vi "GUI_laptop v11c2.vi"() -> ()   [LabVIEW 2019]
uses:
  <vilib>/Math Plots/3D Math Plots/3D Scatter/3D Scatter XCtrl/3D Scatter.xctl
  <vilib>/Platform/TimedLoop/XDataNode/timing_clust.ctl
  <vilib>/Platform/TimedLoop/XDataNode/nitl_modes.ctl
  <vilib>/Platform/TimedLoop/XDataNode/wakeup.ctl
  <vilib>/Analysis/_algsub.llb/Real Vector Norm.vi
  <vilib>/Instr/_visa.llb/VISA Configure Serial Port (Instr).vi
  <vilib>/Utility/file.llb/Write Delimited Spreadsheet (DBL).vi
  <vilib>/Math Plots/3D Math Plots/3D Scatter/3D Scatter Datatype/Public/Plot Helper (Vector).vi
  <vilib>/platform/TimedLoop/XDataNode/XDataNode.xnode
  <vilib>/Platform/TimedLoop/XDataNode/XDNodeRunTimeDep.lvlib
  <vilib>/Analysis/NI_AALPro.lvlib
  <vilib>/Math Plots/3D Math Plots/3D Scatter/3D Scatter Datatype/3D Scatter Datatype.lvclass
panel:
  in  "L5 Scale":dbl=330.0
  in  "L5 Upper Bound":dbl=330.0
  in  "L5 Lower Bound":dbl=320.0
  in  "Motion Scale 4":dbl=2.0
  out "spreadsheet string":string
  out "1-D Array of Real 2":dbl[](array[numeric])
  out "1-D Array of Real":dbl[](array[numeric])
  in  "Save Path 2":path=path "C:/Users/jimmy/Documents/GitHub/Arduino-LabVIEW/zhantao/read_data_delt.csv"
  out "Numeric":i32
  out "send values":dbl[](array[numeric])
  out "Robot Feedback (xyz)":dbl[](array[numeric])
  in  "UDP Send":bool
  in  "UDP Recv":bool
  in  "L5 bound":dbl=1000.0
  in  "L4 bound (deg)":dbl=1000.0
  in  "L3 bound (mm)":dbl=1000.0
  in  "L2 bound (deg)":dbl=1000.0
  in  "L1 bound (deg)":dbl=1000.0
  in  "Joystick Type":dbl(ring) items=["Rigid Joystick", "Free Joystick"]
  out "Finished Late? [i-1]":bool
  in  "Epsilon":dbl=0.2
  out "3D Scatter":refnum<class "3D Plot Datatype.lvclass">[](xcontrol)
  out "Random Point":dbl[](array[numeric])
  out "Virtual Cursor":dbl[](array[numeric])
  out "Iteration Duration":i64
  in  "Num of Points":i32=10
  in  "z bound":dbl=2.0
  in  "y bound":dbl=5.0
  in  "x bound":dbl=5.0
  in  "Stop":bool
  in  "Round Decimals":dbl=2.0 format="%#_15g"
  in  "Save  Data":bool
  in  "Save Path":path=path "C:/Users/jimmy/Documents/GitHub/Arduino-LabVIEW/zhantao/read_data_abs.csv"
  in  "x speed":dbl=0.5
  in  "z speed":dbl=0.5
  in  "y speed":dbl=0.5
  out "error out":errorcluster
  in  "baud rate":u32=115200
  in  "VISA resource name":refnum<visa-resource-name>
  # "TODO: fix the bounds; currently bounds are arbitrary"
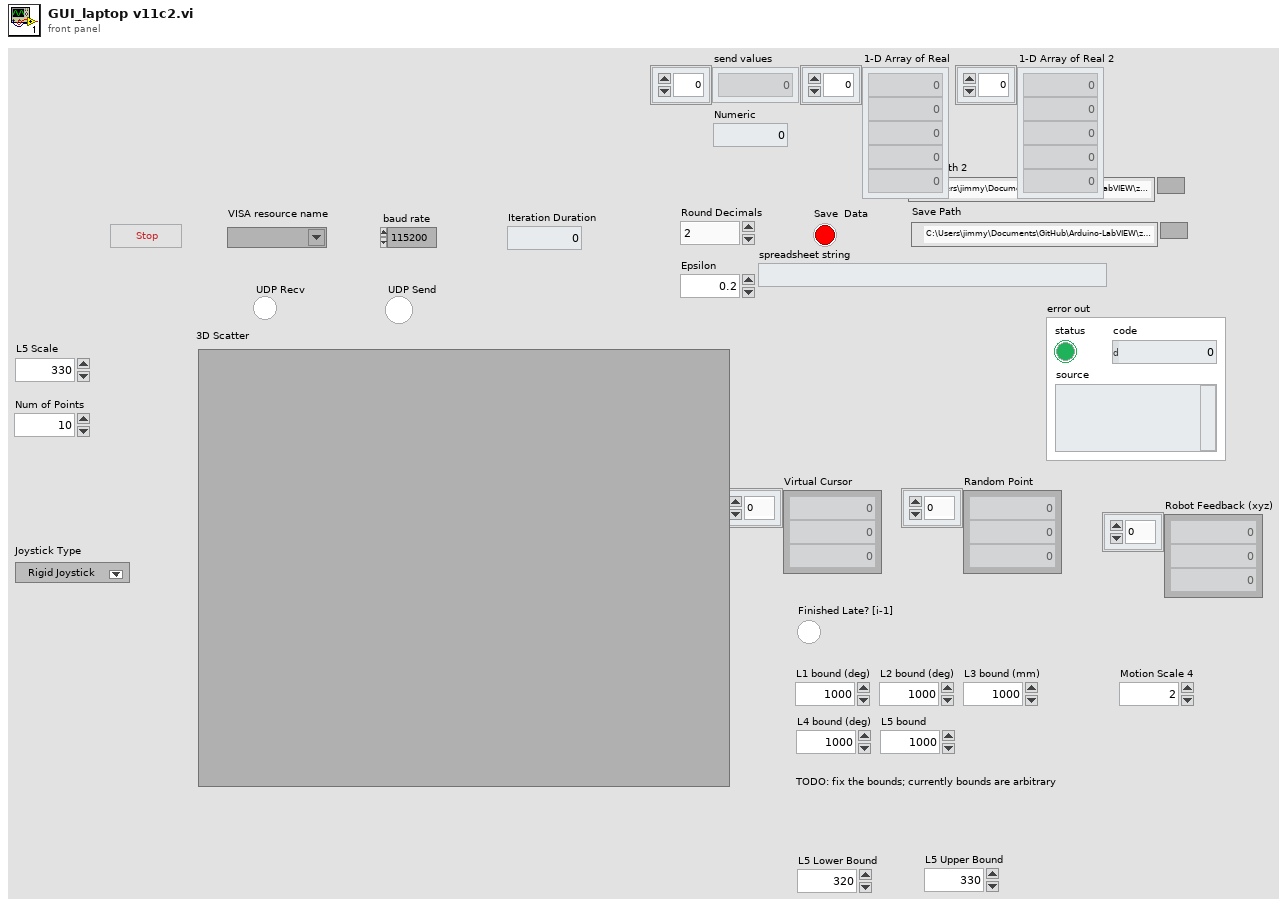
[diagram p1: front panel]
types:
  T1 = typedef "XDNodeRunTimeDep.lvlib/timing_clust.ctl" = cluster{"Expected End [f-1]":u64, "Actual End [f-1]":u64, "Finished Late? [f-1]":bool, "Expected End [i-1]":u64, "Actual End [i-1]":u64, "Finished Late? [i-1]":bool, "Expected Start [i]":u64, "Actual Start [i]":u64, "Expected Start [f]":u64, "Actual Start [f]":u64, "Source Name":string, "Structure Name":string, "Period":i64, "Deadline":i64, "Offset":i64, "Start":i64, "Priority":i32, "Timeout":i32, "Mode":T2, "Wakeup Reason":T3, "Error":errorcluster, "Source Type":string, "Secondary Source Type":string, "Global End Time":u64, "Global Start Time":u64, "Frame Duration":u64, "Iteration Duration":u64, "Assigned CPU":i32, "I/O Scan Engine Mode":u32}
  T2 = typedef "XDNodeRunTimeDep.lvlib/nitl_modes.ctl" = enum32{"No Change", "Process missed periods, maintain original phase", "Discard missed periods, maintain original phase", "Process missed periods, ignore original phase", "Discard missed periods, ignore original phase"}
  T3 = typedef "XDNodeRunTimeDep.lvlib/wakeup.ctl" = enum32{"Normal", "Aborted", "Asynchronous wakeup", "Timing source error", "Timed loop error", "Timeout"}
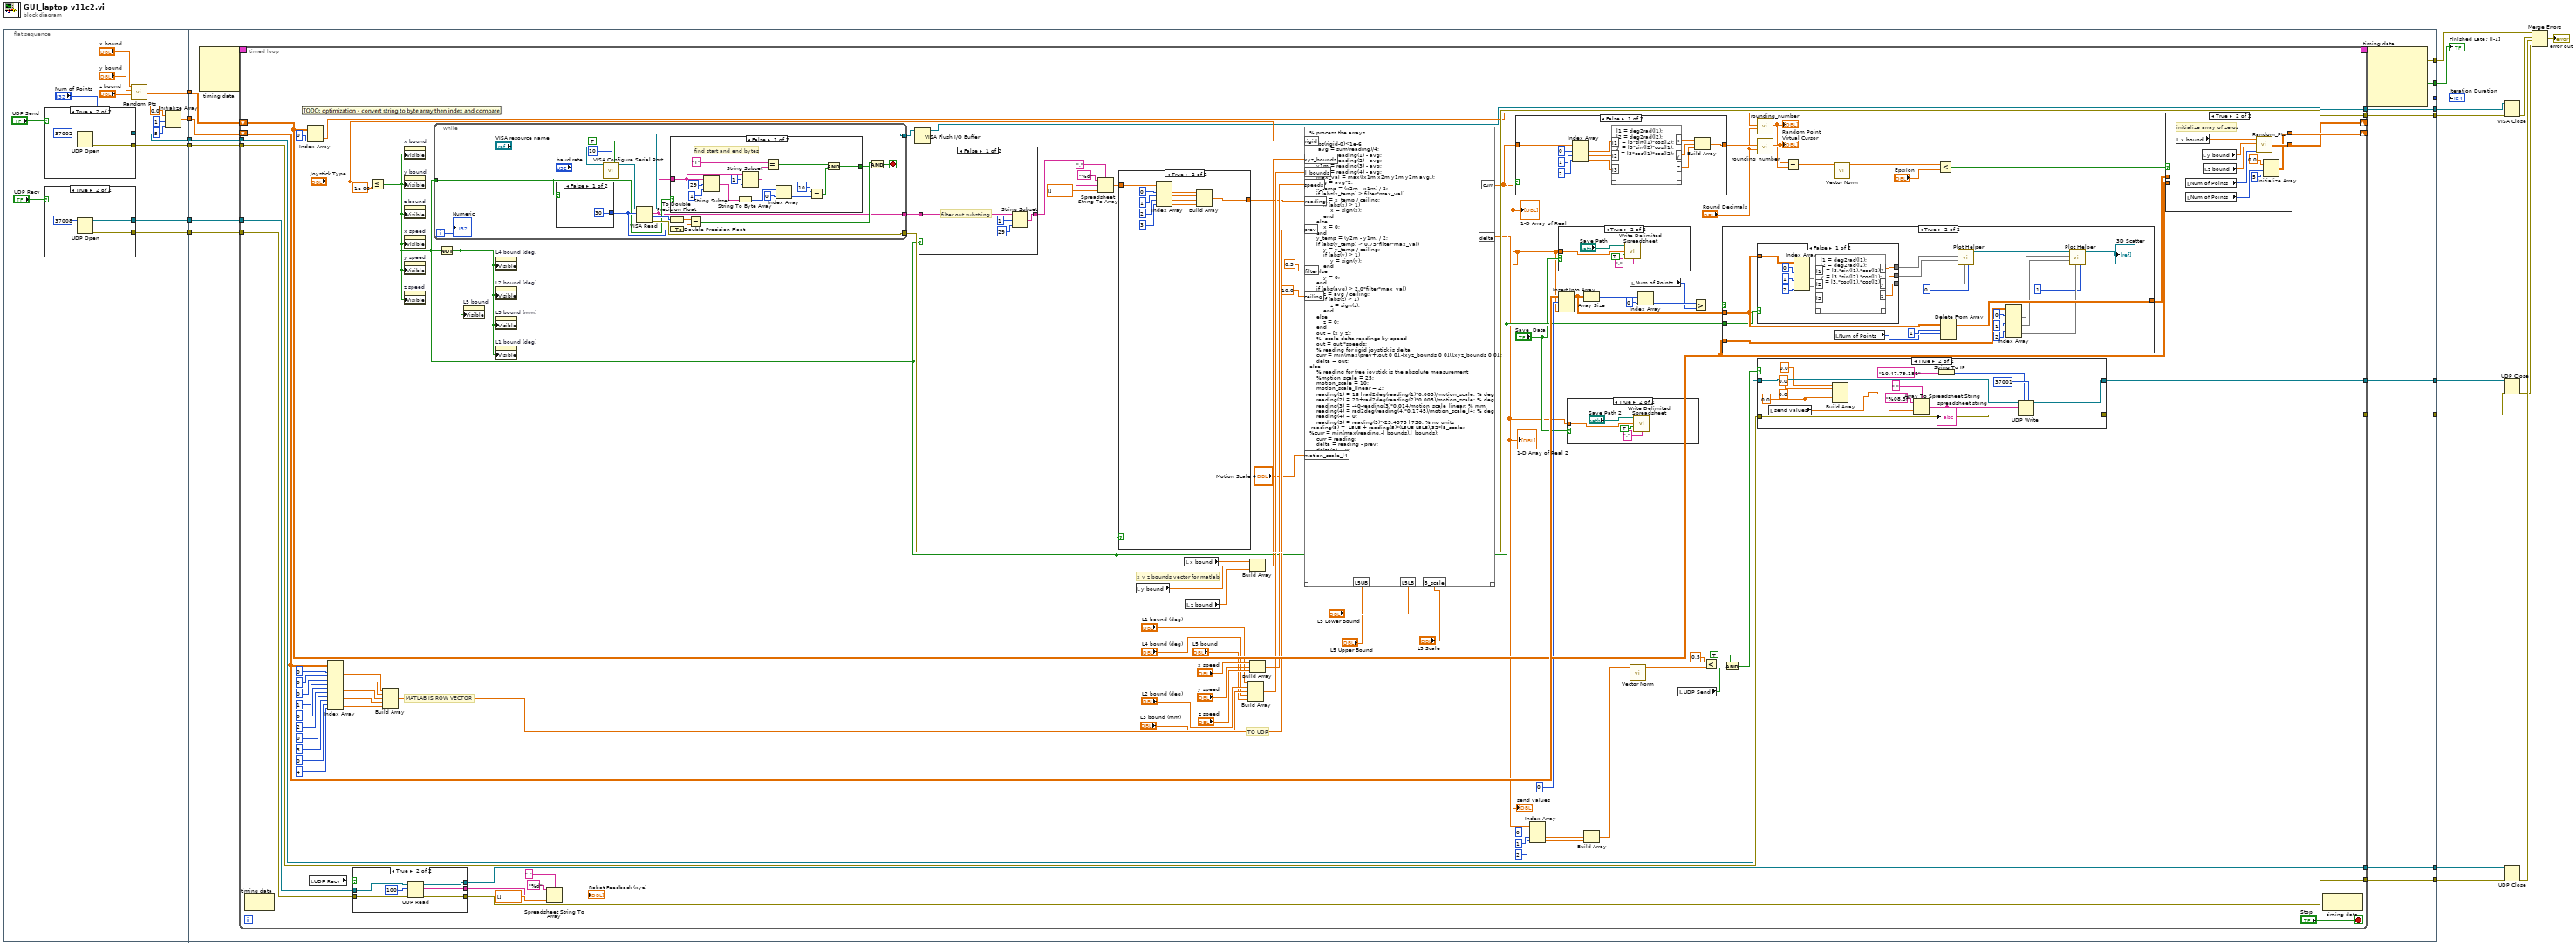
[diagram p0: block diagram]
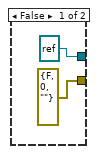
[diagram p2: hidden frame]
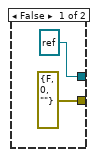
[diagram p3: hidden frame]
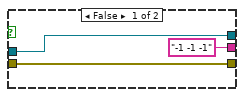
[diagram p6: hidden frame]
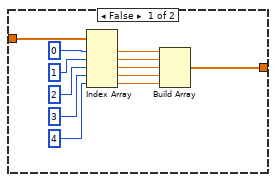
[diagram p10: hidden frame]
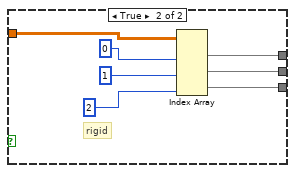
[diagram p13: hidden frame]
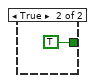
[diagram p14: hidden frame]
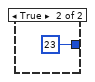
[diagram p15: hidden frame]
diagram:
  n1 = flat-sequence {
    tunnel: [w26] -> w15
    tunnel: [w30] -> w14
    tunnel: [w25] -> w13
    tunnel: [w24] -> w12
    tunnel: [w21] -> w11
    tunnel: [w20] -> w10
    tunnel: [w59] -> w19
    tunnel: [w58] -> w18
    tunnel: [w56] -> w9
    tunnel: [w54] -> w17
    tunnel: [w53] -> w16
    tunnel: w15 -> [w57]
    tunnel: w14 -> [w55]
    tunnel: w13 -> [w52]
    tunnel: w12 -> [w51]
    tunnel: w11 -> [w50]
    tunnel: w10 -> [w49]
    tunnel: [w48] -> w3
    tunnel: [w47] -> w8
    tunnel: [w46] -> w2
    tunnel: [w45] -> w1
    frame #0 {
      n2 = case shown="True" "UDP Send" {
        tunnel: [refnum<k16> refnum ("port") w38] -> w25
        tunnel: [errorcluster {"status"=FALSE, "code"=0, "source"=""} ("error out") w37] -> w20
        frame False {
        }
        frame True {
          n3 = UDP Open(11:u16 37002 ("port")) -> (port=w38:refnum<k16>, 0:w37:errorcluster)  [unwired: 4 in, 1 out]
        }
      }
      n4 = case shown="True" "UDP Recv" {
        tunnel: [refnum<k16> refnum ("port") w43] -> w24
        tunnel: [errorcluster {"status"=FALSE, "code"=0, "source"=""} ("error out") w42] -> w21
        frame False {
        }
        frame True {
          n5 = UDP Open(11:u16 37008 ("port")) -> (port=w43:refnum<k16>, 0:w42:errorcluster)  [unwired: 4 in, 1 out]
        }
      }
      n6 = call "Random_Pts.vi"("Num of Points"="Num of Points", "z bound"="z bound", "y bound"="y bound", "x bound"="x bound") -> ("appended array"=w30:dbl[][])
      n7 = Initialize Array(0.0 ("element"), 1 ("dimension size"), 5 ("dimension size")) -> (w26:dbl[][])
    }
    frame #1 {
      n8 = node-c288() -> (w61:T1)  [unwired: 4 in]
      n9 = timed-loop {
        tunnel: [w70] -> w59
        tunnel: [w162] -> w58
        shift-right: [w161] -> _
        shift-left: w57 -> [w160]
        timing: w61 -> [_]
        timing-out: [_] -> w60
        shift-right: [w156] -> _
        shift-left: w55 -> [w157]
        tunnel: w52 -> [w100]
        tunnel: w51 -> [w99]
        tunnel: w50 -> [w97]
        tunnel: w49 -> [w96]
        tunnel: [w95] -> w48
        tunnel: [w94] -> w47
        tunnel: [w93] -> w46
        tunnel: [w92] -> w45
        stop <- "Stop" stop-if-true
        # "TO UDP"
        # "MATLAB IS ROW VECTOR"
        # "x y z bounds vector for matlab"
        n10 = node-c288() -> ()  [unwired: 1 in, 1 out]
        n11 = Index Array(array=w157, index (col)=0 ("index (row)")) -> (element=w109:dbl[])  [unwired: 1 in]
        n12 = local read "UDP Recv"() -> (w98:bool)
        n13 = Index Array(array=w160, index (row) #1=0 ("disabled index (row)"), index (col) #1=0 ("disabled index (col)"), index (row) #2=0 ("disabled index (row)"), index (col) #2=1 ("disabled index (col)"), index (row) #3=0 ("disabled index (row)"), index (col) #3=2 ("disabled index (col)"), index (row) #4=0 ("disabled index (row)"), index (col) #4=3 ("disabled index (col)"), index (row) #5=0 ("disabled index (row)"), index (col) #5=4 ("disabled index (col)")) -> (element #1=w133:dbl, element #2=w132:dbl, element #3=w131:dbl, element #4=w117:dbl, element #5=w116:dbl)
        n14 = case shown="True" w98 {
          tunnel: w99 -> [w186 w193]
          tunnel: w97 -> [w187 w192]
          tunnel: [w187 w191] -> w95
          tunnel: [w186 w190] -> w93
          tunnel: ["-1 -1 -1" w188] -> w88
          frame False {
          }
          frame True {
            n15 = UDP Read(connection ID=w193, max size (548)=100, 8:w192) -> (data out=w188:string, error out=w191:errorcluster, 3:w190:refnum<k16>)  [unwired: 1 in, 2 out]
          }
        }
        n16 = Less Or Equal?(x="Joystick Type", y=1e-06) -> (x <= y?=w75:bool)
        n17 = Build Array(w133, w132, w131, w117, w116) -> (w130:dbl[])
        n18 = property on="x bound" class="DigNum (strict)"("Visible"=w75) -> ()  [unwired: 2 in, 2 out]
        n19 = property on="y bound" class="DigNum (strict)"("Visible"=w75) -> ()  [unwired: 2 in, 2 out]
        n20 = property on="z bound" class="DigNum (strict)"("Visible"=w75) -> ()  [unwired: 2 in, 2 out]
        n21 = property on="x speed" class="DigNum (strict)"("Visible"=w75) -> ()  [unwired: 2 in, 2 out]
        n22 = property on="y speed" class="DigNum (strict)"("Visible"=w75) -> ()  [unwired: 2 in, 2 out]
        n23 = property on="z speed" class="DigNum (strict)"("Visible"=w75) -> ()  [unwired: 2 in, 2 out]
        n24 = while {
          tunnel: [w286] -> w111
          tunnel: [w299] -> w162
          tunnel: [w293] -> w71
          tunnel: w75 -> [w287]
          i -> [w285]
          stop <- w289 stop-if-true
          n25 = case shown="False" w287 {
            tunnel: [30 u32 23 ("byte count")] -> w292
            frame False {
            }
            frame True {
            }
          }
          n26 = call-poly "VISA Configure Serial Port"("VISA resource name"="VISA resource name", "termination char\n(0xA = '\\n' = LF)"=u8 10 ("termination char\n(0xA = '\\n' = LF)"), "Enable Termination\nChar (T)"=TRUE ("Enable Termination\nChar (T)"), "baud rate (9600)"="baud rate") -> ("VISA resource name out"=w294:refnum<visa-resource-name>)  [unwired: 10 in, 1 out]
          n27 = VISA Read(VISA resource name=w294, byte count=w292) -> (VISA resource name out=w293:refnum<visa-resource-name>, read buffer=w286:string, return count=w301:u32, error out=w299:errorcluster)  [unwired: 1 in]
          n28 = To Double Precision Float(number=w301) -> (double precision float=w300:dbl)
          n29 = To Double Precision Float(number=w292) -> (double precision float=w291:dbl)
          n30 = case shown="False" w287 {
            tunnel: [w308 TRUE] -> w288
            tunnel: w286 -> [w311 _]
            frame False {
              # "find start and end bytes"
              n31 = String Subset(string=w311, offset (0)=29, length (rest)=1) -> (substring=w306:string)
              n32 = String To Byte Array(string=w306) -> (unsigned byte array=w305:u8[])
              n33 = String Subset(string=w311, length (rest)=1) -> (substring=w314:string)  [unwired: 1 in]
              n34 = Equal?(x="T", y=w314) -> (x = y?=w310:bool)
              n35 = Index Array(array=w305, index=0) -> (element=w303:u8)
              n36 = Equal?(x=10, y=w303) -> (x = y?=w309:bool)
              n37 = And(x=w310, y=w309) -> (x .and. y?=w308:bool)
            }
            frame True {
            }
          }
          n38 = Equal?(x=w300, y=w291) -> (x = y?=w290:bool)
          n39 = And(x=w290, y=w288) -> (x .and. y?=w289:bool)
          "Numeric" <- w285
        }
        n40 = Not(x=w75) -> (.not. x?=w74:bool)
        n41 = property on="L5 bound" class="DigNum (strict)"("Visible"=w74) -> ()  [unwired: 2 in, 2 out]
        n42 = property on="L4 bound (deg)" class="DigNum (strict)"("Visible"=w74) -> ()  [unwired: 2 in, 2 out]
        n43 = property on="L2 bound (deg)" class="DigNum (strict)"("Visible"=w74) -> ()  [unwired: 2 in, 2 out]
        n44 = property on="L3 bound (mm)" class="DigNum (strict)"("Visible"=w74) -> ()  [unwired: 2 in, 2 out]
        n45 = property on="L1 bound (deg)" class="DigNum (strict)"("Visible"=w74) -> ()  [unwired: 2 in, 2 out]
        n46 = Spreadsheet String To Array(delimiter (Tab)=" ", format string="%d", spreadsheet string=w88, array type (2D Dbl)=dbl[] []) -> (array=→"Robot Feedback (xyz)":dbl[])
        n47 = VISA Flush I/O Buffer(VISA resource name=w71) -> (VISA resource name out=w70:refnum<visa-resource-name>)  [unwired: 2 in, 1 out]
        n48 = case shown="False" w75 {
          tunnel: w111 -> [w212 w213]
          tunnel: [w209 w213] -> w110
          frame False {
            # "filter out substring"
            n49 = String Subset(string=w212, offset (0)=1, length (rest)=29) -> (substring=w209:string)
          }
          frame True {
          }
        }
        n50 = Spreadsheet String To Array(delimiter (Tab)=",", format string="%d", spreadsheet string=w110, array type (2D Dbl)=dbl[] []) -> (array=w113:dbl[])
        n51 = case shown="True" w75 {
          tunnel: w113 -> [w214 w229]
          tunnel: [w219 w228] -> w112
          frame False {
            n52 = Index Array(array=w214, index #1=0 ("Plot ID"), index #2=1 ("Plot ID"), index #3=2 ("Plot ID"), index #4=3 ("Plot ID"), index #5=4 ("Plot ID")) -> (element #1=w222:dbl, element #2=w221:dbl, element #3=w220:dbl, element #4=w216:dbl, element #5=w215:dbl)
            n53 = Build Array(w222, w221, w220, w216, w215) -> (w219:dbl[])
          }
          frame True {
            n54 = Index Array(array=w229, index #1=0 ("Plot ID"), index #2=1 ("Plot ID"), index #3=2 ("Plot ID"), index #4=3 ("index")) -> (element #1=w232:dbl, element #2=w231:dbl, element #3=w230:dbl, element #4=w226:dbl)
            n55 = Build Array(w232, w231, w230, w226) -> (w228:dbl[])
          }
        }
        n56 = local read "y bound"() -> (w135:dbl)
        n57 = local read "x bound"() -> (w136:dbl)
        n58 = local read "z bound"() -> (w134:dbl)
        n59 = Build Array("L1 bound (deg)", "L2 bound (deg)", "L3 bound (mm)", "L4 bound (deg)", "L5 bound") -> (w124:dbl[])
        n60 = Build Array(w136, w135, w134) -> (w128:dbl[])
        n61 = Build Array("x speed", "y speed", "z speed") -> (w129:dbl[])
        n62 = script code="% process the arrays\n\nif abs(rigid-0)<1e-6\n     avg = sum(reading)/4;\n    x1m = reading(1) - avg;\n    x2m = reading(2) - avg;\n    y1m = reading(3) - avg;\n    y2m = reading(4) - avg;\n    max_val = max([x1m x2m y1m y2m avg]);\n    avg = avg*2;\n    x_temp = (x2m - x1m) / 2;\n    if (abs(x_temp) > filter*max_val)\n        x = x_temp / ceiling;\n        if (abs(x) > 1)\n            x = sign(x);\n        end\n    else\n        x = 0;\n    end\n    y_temp = (y2m - y1m) / 2;\n    if (abs(y_temp) > 0.75*filter*max_val)\n        y = y_temp / ceiling;\n        if (abs(y) > 1)\n            y = sign(y);\n        end\n    else\n        y = 0;\n    end\n    if (abs(avg) > 2.0*filter*max_val)\n        z = avg / ceiling;\n        if (abs(z) > 1)\n            z = sign(z);\n        end\n    else\n        z = 0;\n    end\n    out = [x y z];\n    %  scale delta readings by speed\n    out = out.*speeds;\n    % reading for rigid joystick is delta\n    curr = min(max(prev+[out 0 0],-[xyz_bounds 0 0]),[xyz_bounds 0 0]);\n    delta = out;\nelse\n    % reading for free joystick is the absolute measurement\n    %motion_scale = 25;\n    motion_scale = 10;\n    motion_scale_linear = 2;\n    reading(1) = 16+rad2deg(reading(1)*0.005)/motion_scale; % deg\n    reading(2) = 20+rad2deg(reading(2)*0.005)/motion_scale; % deg\n    reading(3) = -40-reading(3)*0.014/motion_scale_linear; % mm\n    reading(4) = rad2deg(reading(4)*0.1745)/motion_scale_l4; % deg\n    reading(4) = 0;\n    reading(5) = reading(5)*-23.4375+750; % no units\n reading(5) =  L5LB + reading(5)*(L5UB-L5LB)/32*l5_scale;\n%curr = min(max(reading,-l_bounds),l_bounds);\n    curr = reading;\n    delta = reading - prev;\n    delta(5) = 0;\nend"("xyz_bounds"=w128, "speeds"=w129, "reading"=w112, "prev"=w130, "rigid"="Joystick Type", "l_bounds"=w124, "filter"=0.3 ("Real"), "ceiling"=10.0 ("Real"), "motion_scale_l4"="Motion Scale 4", "L5UB"="L5 Upper Bound", "L5LB"="L5 Lower Bound", "l5_scale"="L5 Scale") -> ("curr"=w66:dbl[], "delta"=w67:dbl[])  [unwired: 1 in, 1 out]
        "send values" <- w66
        "1-D Array of Real" <- w66
        "1-D Array of Real 2" <- w67
        n63 = case shown="False" w75 {
          tunnel: w66 -> [w243 w247]
          tunnel: [w236 w247] -> w158
          frame False {
            n64 = Index Array(array=w243, index #1=0 ("Plot ID"), index #2=1 ("Plot ID"), index #3=2 ("Plot ID")) -> (element #1=w242:dbl, element #2=w241:dbl, element #3=w240:dbl)
            n65 = script code="l1 = deg2rad(l1);\nl2 = deg2rad(l2);\nx = l3*sin(l1)*cos(l2);\ny = l3*sin(l2)*cos(l1);\nz = l3*cos(l1)*cos(l2);"("l1"=w242, "l2"=w241, "l3"=w240) -> ("x"=w239:dbl, "y"=w238:dbl, "z"=w237:dbl)  [unwired: 1 in, 1 out]
            n66 = Build Array(w239, w238, w237) -> (w236:dbl[])
          }
          frame True {
          }
        }
        n67 = Index Array(array=w67, index #1=0 ("disabled index (col)"), index #2=1 ("disabled index (col)"), index #3=2 ("disabled index (col)")) -> (element #1=w79:dbl, element #2=w78:dbl, element #3=w77:dbl)
        n68 = case shown="True" "Save  Data" {
          tunnel: w66 -> [_ w195]
          frame False {
          }
          frame True {
            n69 = call-poly <vilib>:"Write Delimited Spreadsheet.vi"("file path (dialog if empty)"="Save Path", "1D data"=w195, "append to file? (new file:F)"=TRUE, "delimiter (\\t)"="," ("delimiter (\\t)")) -> ()  [unwired: 10 in, 2 out]
          }
        }
        n70 = Insert Into Array(array=w160, index (row)=0, new element=w66) -> (w141:dbl[][])  [unwired: 1 in]
        n71 = case shown="True" "Save  Data" {
          tunnel: w67 -> [_ w165]
          frame False {
          }
          frame True {
            n72 = call-poly <vilib>:"Write Delimited Spreadsheet.vi"("file path (dialog if empty)"="Save Path 2", "1D data"=w165, "append to file? (new file:F)"=TRUE, "delimiter (\\t)"="," ("delimiter (\\t)")) -> ()  [unwired: 10 in, 2 out]
          }
        }
        n73 = Array Size(array=w141) -> (size(s)=w143:i32[])
        n74 = Build Array(w79, w78, w77) -> (w76:dbl[])
        n75 = local read "Num of Points"() -> (w142:i32)
        n76 = call-poly <vilib>:"Vector Norm.vi"("Input Vector"=w76) -> ("norm"=w86:dbl)  [unwired: 9 in, 1 out]
        n77 = Index Array(array=w143, index=0) -> (element=w144:i32)
        n78 = local read "UDP Send"() -> (w84:bool)
        n79 = Greater?(x=w144, y=w142) -> (0:w140:bool)
        n80 = Less?(x=0.5, y=w86) -> ()  [unwired: 1 out]
        n81 = case shown="True" w140 {
          tunnel: w141 -> [w248 w266]
          tunnel: [w248 w265] -> w159
          tunnel: w157 -> [_ w264]
          tunnel: w75 -> [_ w249]
          frame False {
          }
          frame True {
            n82 = case shown="False" w249 {
              tunnel: w266 -> [w277 w281]
              tunnel: [w268 w280] -> w255
              tunnel: [w269 w279] -> w254
              tunnel: [w270 w278] -> w253
              frame False {
                n83 = Index Array(array=w277, index (col) #1=0 ("Plot ID"), index (col) #2=1 ("Plot ID"), index (col) #3=2 ("Plot ID")) -> (element #1=w273:dbl[], element #2=w272:dbl[], element #3=w271:dbl[])  [unwired: 3 in]
                n84 = script code="l1 = deg2rad(l1);\nl2 = deg2rad(l2);\nx = l3.*sin(l1).*cos(l2);\ny = l3.*sin(l2).*cos(l1);\nz = l3.*cos(l1).*cos(l2);"("l1"=w273, "l2"=w272, "l3"=w271) -> ("x"=w268:dbl[], "y"=w269:dbl[], "z"=w270:dbl[])  [unwired: 1 in, 1 out]
              }
              frame True {
                # "rigid"
                n85 = Index Array(array=w281, index (col) #1=0 ("disabled index (col)"), index (col) #2=1 ("index (col)"), index (col) #3=2 ("index (col)")) -> (element #1=w280:dbl[], element #2=w279:dbl[], element #3=w278:dbl[])  [unwired: 3 in]
              }
            }
            n86 = local read "Num of Points"() -> (w263:i32)
            n87 = Delete From Array(array=w266, length=1, index (row)=w263) -> (array with subset deleted=w265:dbl[][])  [unwired: 1 in, 1 out]
            n88 = call-poly <vilib>:"Plot Helper.vi"("Plot ID"=0, "z vector"=w253, "y vector"=w254, "x vector"=w255) -> ("3D Plot lvclass Array out"=w257:refnum<class "3D Plot Datatype.lvclass">[])  [unwired: 2 in, 5 out]
            n89 = Index Array(array=w264, index (row) #1=0 ("index (row)"), index (row) #2=1 ("index (row)"), index (row) #3=2 ("index (row)")) -> (element #1=w261:dbl[], element #2=w260:dbl[], element #3=w259:dbl[])  [unwired: 3 in]
            n90 = call-poly <vilib>:"Plot Helper.vi"("Plot ID"=1, "z vector"=w259, "y vector"=w260, "x vector"=w261, "3D Plot lvclass Array in"=w257) -> ("3D Plot lvclass Array out"=→"3D Scatter":refnum<class "3D Plot Datatype.lvclass">[])  [unwired: 1 in, 5 out]
          }
        }
        n91 = And(x=TRUE, y=w84) -> (x .and. y?=w83:bool)
        n92 = call "rounding_number.vi"("power of ten"="Round Decimals", "Array"=w109) -> ("rounded"=w106:dbl[])  [unwired: 9 in]
        "Random Point" <- w106
        n93 = call "rounding_number.vi"("power of ten"="Round Decimals", "Array"=w158) -> ("rounded"=w107:dbl[])  [unwired: 9 in]
        "Virtual Cursor" <- w107
        n94 = case shown="True" w83 {
          tunnel: w100 -> [w168 w184]
          tunnel: w96 -> [w169 w180]
          tunnel: [w169 w176] -> w94
          tunnel: [w168 w175] -> w92
          frame False {
          }
          frame True {
            w174 = 0.0 ("element")
            n95 = local read "send values"() -> (w170:dbl[])
            n96 = Build Array(0.0 ("element"), 0.0 ("element"), 0.0 ("element"), w174, w174) -> ()  [unwired: 1 out]
            n97 = Array To Spreadsheet String(delimiter (Tab)=" ", array=w170, 3:"%08.3f" ("format string")) -> (spreadsheet string=w181:string)
            "spreadsheet string" <- w181
            n98 = String To IP(1:"10.47.79.181" ("name")) -> (0:w178:u32)
            n99 = UDP Write(address=w178, port or service name=u16 37001, connection ID=w184, data in=w181, 8:w180) -> (error out=w176:errorcluster, 3:w175:refnum<k16>)  [unwired: 1 in]
          }
        }
        n100 = Subtract(x=w107, y=w106) -> (x-y=w105:dbl[])
        n101 = call-poly <vilib>:"Vector Norm.vi"("Input Vector"=w105) -> ("norm"=w104:dbl)  [unwired: 9 in, 1 out]
        n102 = Less?(x=w104, y="Epsilon") -> (x < y?=w102:bool)
        n103 = case shown="True" w102 {
          tunnel: w157 -> [w199 _]
          tunnel: [w199 w204] -> w156
          tunnel: w159 -> [w198 _]
          tunnel: [w198 w200] -> w161
          frame False {
          }
          frame True {
            # "initialize array of zeros"
            n104 = local read "x bound"() -> (w208:dbl)
            n105 = local read "Num of Points"() -> (w205:i32)
            n106 = local read "Num of Points"() -> (w202:i32)
            n107 = local read "y bound"() -> (w207:dbl)
            n108 = local read "z bound"() -> (w206:dbl)
            n109 = call "Random_Pts.vi"("Num of Points"=w205, "z bound"=w206, "y bound"=w207, "x bound"=w208) -> ("appended array"=w204:dbl[][])
            n110 = Initialize Array(0.0 ("element"), w202, 5 ("dimension size")) -> (w200:dbl[][])
          }
        }
        n111 = node-c288() -> ()  [unwired: 1 in, 1 out]
      }
      n112 = node-c288(w60) -> (w56:errorcluster, w53:bool, w54:i64)  [unwired: 3 out]
    }
  }
  n113 = VISA Close(VISA resource name=w19, error in (no error)=w18) -> (error out=w7:errorcluster)
  n114 = UDP Close(connection ID=w1, 8:w8) -> (error out=w5:errorcluster)  [unwired: 1 out]
  n115 = UDP Close(connection ID=w2, 8:w3) -> (error out=w6:errorcluster)  [unwired: 1 out]
  n116 = Merge Errors(w9, w7, w6, w5) -> (→"error out":errorcluster)
  "Iteration Duration" <- w17
  "Finished Late? [i-1]" <- w16
